vi "SwerveOdometry_New.vi"(9 "InitialPose":T4={"TRANSLATION"={"X"=0.0, "Y"=0.0}, "ROTATION"={"VALUE"=0.0, "COS"=1.0, "SIN"=0.0}} {"ROTATION"."SIN" format="%13.4f"; "ROTATION"."COS" format="%13.4f"; "ROTATION"."VALUE" format="%13.4f"; "TRANSLATION"."Y" format="%14.3f"; "TRANSLATION"."X" format="%14.3f"}, 10 "Module Positions":T1[](array[typedef]) {"Angle"."SIN" format="%13.4f"; "Angle"."COS" format="%13.4f"; "Angle"."VALUE" format="%13.4f"}, 11 "GyroAngle":T2={"VALUE"=0.0, "COS"=1.0, "SIN"=0.0} {"SIN" format="%13.4f"; "COS" format="%13.4f"; "VALUE" format="%13.4f"}) -> (3 "SWERVE_DRIVE_ODOMETRY Out":T3={"POSE"={"TRANSLATION"={"X"=0.0, "Y"=0.0}, "ROTATION"={"VALUE"=0.0, "COS"=1.0, "SIN"=0.0}}, "GyroOffset"={"VALUE"=0.0, "COS"=1.0, "SIN"=0.0}, "PreviousAngle"={"VALUE"=0.0, "COS"=1.0, "SIN"=0.0}, "PrevTime"=0.0, "PrevModulePosition"=[], "NumModules"=0} {"PrevModulePosition"."Angle"."SIN" format="%13.4f"; "PrevModulePosition"."Angle"."COS" format="%13.4f"; "PrevModulePosition"."Angle"."VALUE" format="%13.4f"; "PreviousAngle"."SIN" format="%13.4f"; "PreviousAngle"."COS" format="%13.4f"; "PreviousAngle"."VALUE" format="%13.4f"; "GyroOffset"."SIN" format="%13.4f"; "GyroOffset"."COS" format="%13.4f"; "GyroOffset"."VALUE" format="%13.4f"; "POSE"."ROTATION"."SIN" format="%13.4f"; "POSE"."ROTATION"."COS" format="%13.4f"; "POSE"."ROTATION"."VALUE" format="%13.4f"; "POSE"."TRANSLATION"."Y" format="%14.3f"; "POSE"."TRANSLATION"."X" format="%14.3f"})   [LabVIEW 2020, in "Swerve_Odometry_SEN.lvlib"]
doc: "Constructs a SwerveDriveOdometry object.\n \nParameters:\n - gyroAngle The angle reported by the gyroscope.\n - ModulePostions -- Array of module positions (distances)\n - initialPose The starting position of the robot on the field.\n\nReturns\n - SwerveDriveOdometry - Data Structure"
uses:
  Swerve_Odometry_SEN.lvlib
  Cluster_ROTATION2D.ctl
  Cluster_POSE2D.ctl
  Cluster_TRANSLATION2D.ctl
  Cluster_SWERVE_DRIVE_ODOMETRY.ctl
  Cluster_SWERVE_DRIVE_MODULE_POSITION.ctl
  Rotation2D_Get Inverse.vi
  Rotation2D_Combine.vi
  Rotation2d_CreateAngle.vi
  XY to Rotation2d.vi
  Calculate Distance XY.vi
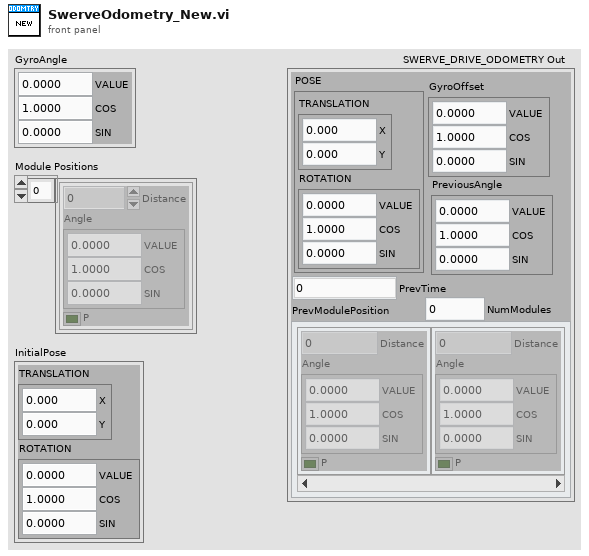
[diagram p1: front panel]
types:
  T1 = typedef "Swerve_Odometry_SEN.lvlib/Cluster_SWERVE_DRIVE_MODULE_POSITION.ctl" = cluster{"Distance":dbl, "Angle":T2, "P":bool}
  T2 = typedef "Swerve_Odometry_SEN.lvlib/Cluster_ROTATION2D.ctl" = cluster{"VALUE":dbl, "COS":dbl, "SIN":dbl}
  T3 = typedef "Swerve_Odometry_SEN.lvlib/Cluster_SWERVE_DRIVE_ODOMETRY.ctl" = cluster{"POSE":T4, "GyroOffset":T2, "PreviousAngle":T2, "PrevTime":dbl, "PrevModulePosition":T1[], "NumModules":i32}
  T4 = typedef "Swerve_Odometry_SEN.lvlib/Cluster_POSE2D.ctl" = cluster{"TRANSLATION":T5, "ROTATION":T2}
  T5 = typedef "Swerve_Odometry_SEN.lvlib/Cluster_TRANSLATION2D.ctl" = cluster{"X":dbl, "Y":dbl}
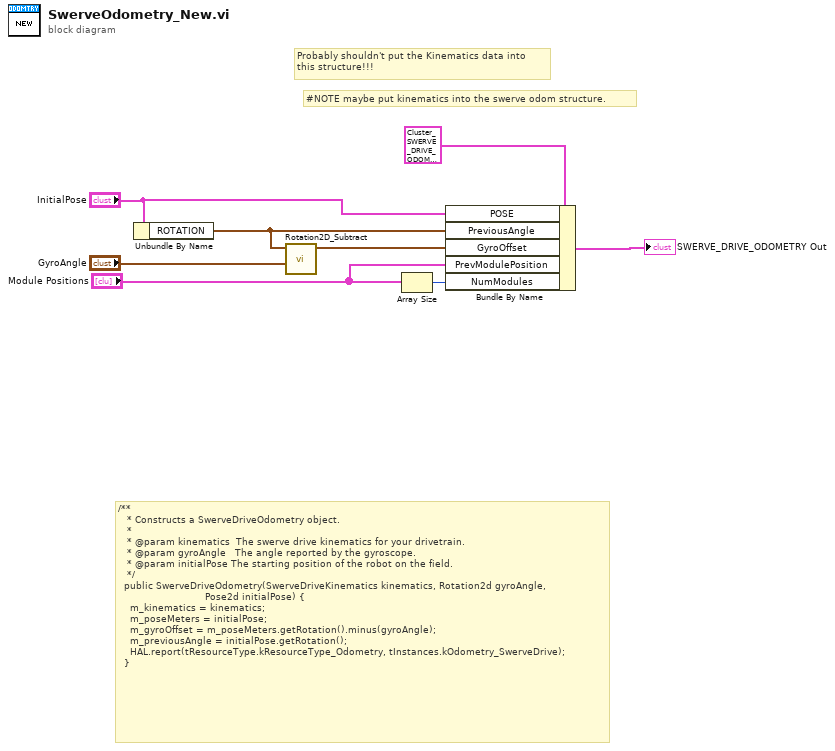
[diagram p0: block diagram]
diagram:
  # "#NOTE maybe put kinematics into the swerve odom structure."
  # "Probably shouldn't put the Kinematics data into\nthis structure!!!"
  # "/**\n   * Constructs a SwerveDriveOdometry object.\n   *\n   * @param kinematics  The swerve drive kinematics for your drivetrain.\n   * @param gyroAngle   The angle reported by the gyroscope.\n   * @param initialPose The starting position of the robot on the field.\n   */\n  public SwerveDriveOdometry(SwerveDriveKinematics kinematics, Rotation2d gyroAngle,\n                             Pose2d initialPose) {\n    m_kinematics = kinematics;\n    m_poseMeters = initialPose;\n    m_gyroOffset = m_poseMeters.getRotation().minus(gyroAngle);\n    m_previousAngle = initialPose.getRotation();\n    HAL.report(tResourceType.kResourceType_Odometry, tInstances.kOdometry_SwerveDrive);\n  }"
  n1 = Unbundle By Name("InitialPose") -> ("ROTATION"=w2:T2)
  n2 = call "Rotation2D_Subtract.vi"("Other ROTATION"="GyroAngle", "In ROTATION"=w2) -> ("Out ROTATION Out"=w6:T2)  [unwired: 9 in]
  n3 = Array Size(array="Module Positions") -> (size(s)=w5:i32)
  n4 = Bundle By Name(cluster=T3 {"POSE"={"TRANSLATION"={"X"=0.0, "Y"=0.0}, "ROTATION"={"VALUE"=0.0, "COS"=1.0, "SIN"=0.0}}, "GyroOffset"={"VALUE"=0.0, "COS"=1.0, "SIN"=0.0}, "PreviousAngle"={"VALUE"=0.0, "COS"=1.0, "SIN"=0.0}, "PrevTime"=0.0, "PrevModulePosition"=[], "NumModules"=0} ("SWERVE_DRIVE_ODOMETRY Out"), "POSE"="InitialPose", "PreviousAngle"=w2, "GyroOffset"=w6, "PrevModulePosition"="Module Positions", "NumModules"=w5) -> (→"SWERVE_DRIVE_ODOMETRY Out":T3)
